vi "ClassParser.vi"(1 "Mode":enum16{"File system", "Project system"}(ring)=enum."Project system", 2 "LabVIEW Object":refnum<class>) -> (0 "TreeItems[]":T1(array[cluster]))   [LabVIEW 2021, in "Tree.lvlib" / "Tree.lvclass"]
uses:
  Tree.lvclass
  Tree.lvclass/Tree.ctl
panel:
  out "Method Paths":path[](array[path])
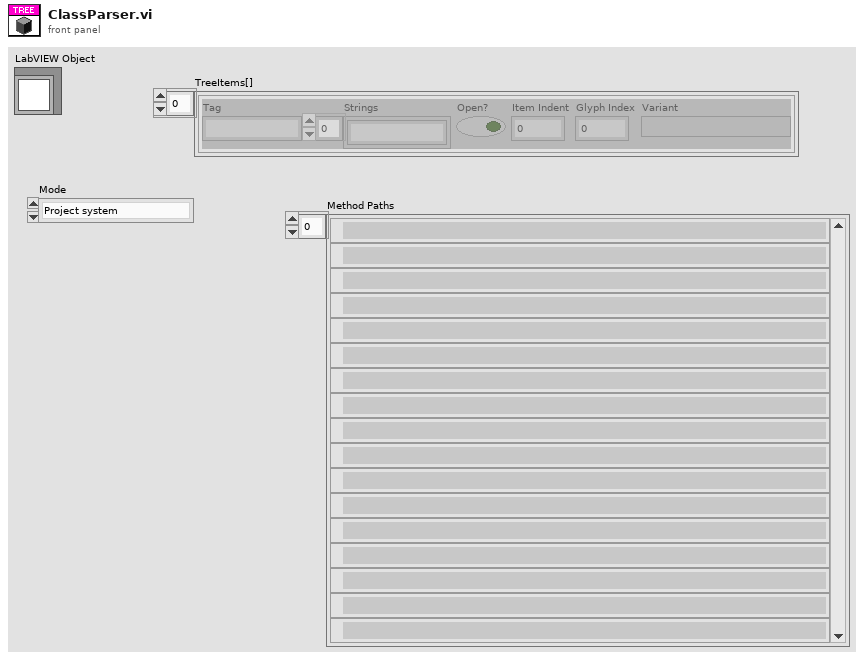
[diagram p1: front panel]
types:
  T1 = cluster{"Tag":string, "Strings":string[], "Open?":bool, "Item Indent":i32, "Glyph Index":i32, "Variant":variant}[]
  T2 = enum32{"invalid scope", "public", "private", "protected", "community"}[]
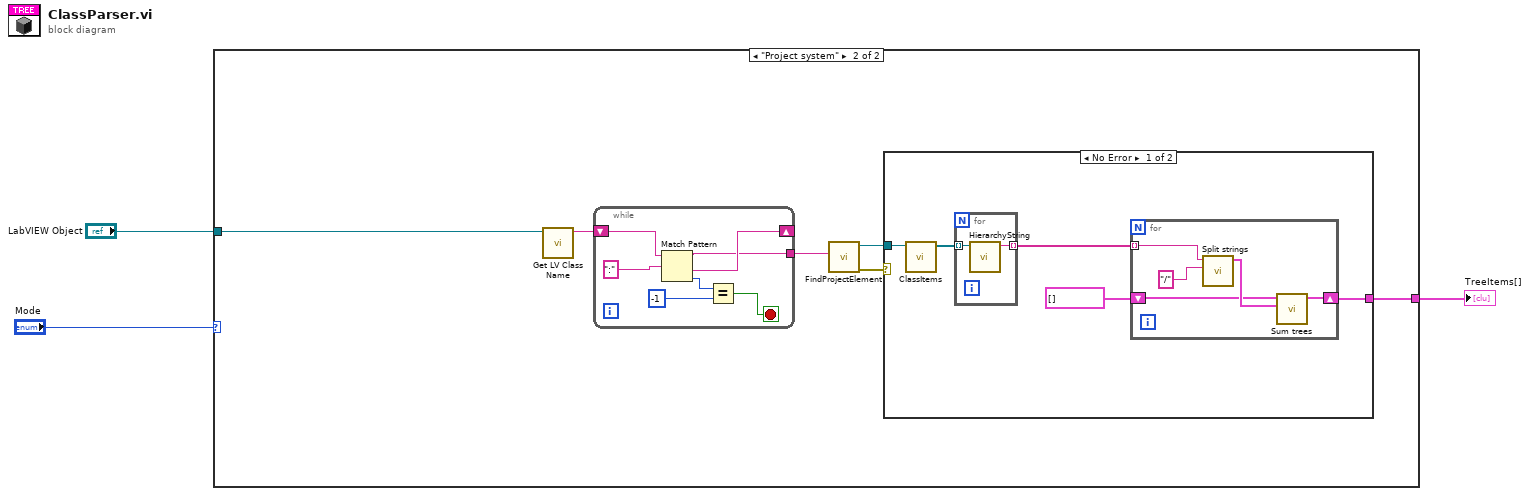
[diagram p0: block diagram]
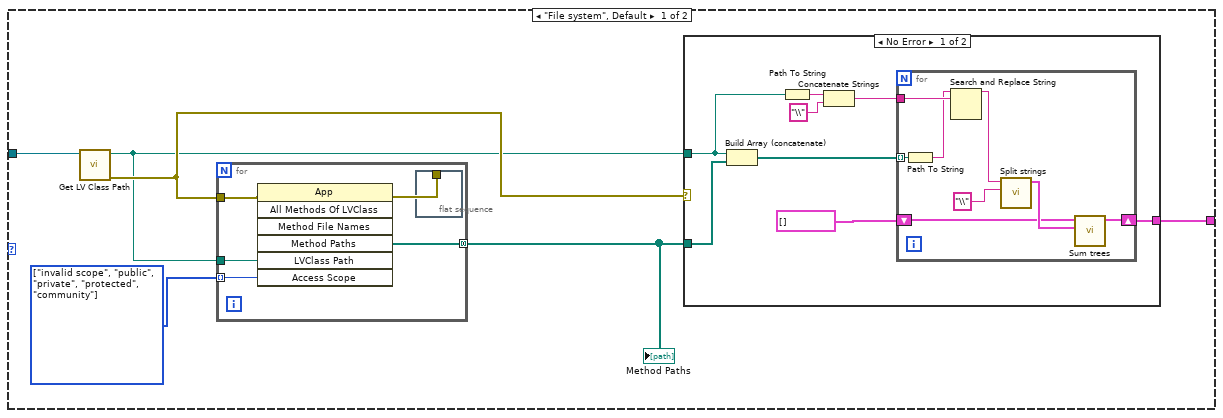
[diagram p2: hidden frame]
diagram:
  n1 = case shown="\"Project system\"" "Mode" {
    tunnel: "LabVIEW Object" -> [w9 w33]
    tunnel: [w7 w32] -> w1
    frame "File system", Default {
      w6 = T2 [enum."invalid scope", enum."public", enum."private", enum."protected", enum."community"] items=["invalid scope", "public", "private", "protected", "community"] ("Access Scope")
      n2 = call <vilib>:"Get LV Class Path.vi"("object"=w9) -> ("error out"=w5:errorcluster, "class path"=w4:path)  [unwired: 9 in]
      n3 = for {
        tunnel: [w14] -> w8 mode=concatenating
        tunnel: w4 -> [w13]
        tunnel: w6 -> [w12] mode=indexing
        tunnel: w5 -> [w11]
        n4 = invoke class="App" method="All Methods Of LVClass"(error in=w11, "LVClass Path"=w13, "Access Scope"=w12) -> (error out=w10:errorcluster, "Method Paths"=w14:path[])  [unwired: 4 in, 5 out]
        n5 = flat-sequence {
          tunnel: w10 -> [_]
          frame #0 {
          }
        }
      }
      "Method Paths" <- w8
      n6 = case shown="No Error" w5 {
        tunnel: w8 -> [w19 _]
        tunnel: w4 -> [w17 _]
        tunnel: [w16 _] -> w7
        frame No Error {
          n7 = Build Array (concatenate)(w17, w19) -> (w18:path[])
          n8 = Path To String(path=w17) -> (string=w20:string)
          n9 = Concatenate Strings(w20, "\\" ("regular expression")) -> (w21:string)
          n10 = for {
            shift-right: [w28] -> w16
            shift-left: T1 [] ("TreeItems[]") -> [w27]
            tunnel: w18 -> [w26] mode=indexing
            tunnel: w21 -> [w25]
            n11 = Path To String(path=w26) -> (string=w24:string)
            n12 = Search and Replace String(input string=w24, search string=w25) -> (result string=w23:string)  [unwired: 6 in, 3 out]
            n13 = call "Split strings.vi"("regular expression"="\\", "qualified name"=w23) -> ("TreeItems[]"=w29:T1)  [unwired: 9 in]
            n14 = call "Sum trees.vi"("Add_to_tree[]"=w29, "TreeItems[]"=w27) -> ("Tree_Out[]"=w28:T1)  [unwired: 9 in]
          }
        }
        frame Error {
        }
      }
    }
    frame "Project system" {
      n15 = call <vilib>:"Get LV Class Name.vi"("object"=w33) -> ("class name"=w34:string)  [unwired: 9 in, 1 out]
      n16 = while {
        shift-right: [w50] -> _
        shift-left: w34 -> [w53]
        tunnel: [w49] -> w35
        stop <- w54 stop-if-true
        n17 = Match Pattern(string=w53, regular expression=":" ("search string/char (-)")) -> (before substring=w49:string, after substring=w50:string, offset past match=w51:i32)  [unwired: 1 in, 1 out]
        n18 = Equal?(x=w51, y=-1) -> (x = y?=w54:bool)
      }
      n19 = call "FindProjectElement.vi"("Element name"=w35) -> ("Error"=w31:errorcluster, "Element out"=w36:refnum<vi>)  [unwired: 8 in, 1 out]
      n20 = case shown="No Error" w31 {
        tunnel: w36 -> [w40 _]
        tunnel: [w38 _] -> w32
        frame No Error {
          n21 = call "ClassItems.vi"("ProjectItem in"=w40) -> ("Owned Items[]"=w41:refnum<vi>[])  [unwired: 10 in]
          n22 = for {
            tunnel: w41 -> [w48] mode=indexing
            tunnel: [w47] -> w39 mode=indexing
            n23 = call "HierarchyString.vi"("ProjectItem"=w48) -> ("Project Path"=w47:string)  [unwired: 9 in, 1 out]
          }
          n24 = for {
            shift-right: [w44] -> w38
            shift-left: T1 [] ("TreeItems[]") -> [w43]
            tunnel: w39 -> [w42] mode=indexing
            n25 = call "Split strings.vi"("regular expression"="/", "qualified name"=w42) -> ("TreeItems[]"=w45:T1)  [unwired: 9 in]
            n26 = call "Sum trees.vi"("Add_to_tree[]"=w45, "TreeItems[]"=w43) -> ("Tree_Out[]"=w44:T1)  [unwired: 9 in]
          }
        }
        frame Error {
        }
      }
    }
  }
  "TreeItems[]" <- w1
